vi "PowerGenerated.vi"() -> ()   [LabVIEW 2009]
uses:
  SubVis/Location.ctl
  <vilib>/Utility/file.llb/Read From Spreadsheet File (DBL).vi
  <vilib>/Analysis/NI_AALBase.lvlib
panel:
  out "Day of Max Power":i32 caption="Day:"
  out "Max Power":dbl caption="Max Power:" format="%#_3pW"
  in  "Location":T1
  out "Max Power (watts)":dbl(slide) caption="2.1MW" scale=0.0..40000000.0 scale format="%#_6pW"
  in  "Stop":bool
  in  "USA":bool
  in  "CostaRica":bool
  in  "Brazil":bool
  in  "India":bool
  in  "Australia":bool
  in  "Japan":bool
  in  "SouthAfrica":bool
  in  "Israel":bool
  in  "Germany":bool
  in  "Days of Month":u8(slide)=30 min=1 max=30 step=1 scale=1.0..30.0
  out "USA_Select":u16(ring)
  out "Germany_Select":u16(ring)
  out "Brazil_Select":u16(ring)
  out "Israel_Select":u16(ring)
  out "India_Select":u16(ring)
  out "Japan_Select":u16(ring)
  out "SouthAfrica_Select":u16(ring)
  out "Australia_Select":u16(ring)
  out "CostaRica_Select":u16(ring)
  out "Wind Speed of All Countries":waveform(dbl)[](graph)
  out "Power Per Country":dbl[](graph)
  # "The day of maximum power output for a given location is determined for all days starting from the first day of the month until the selected day. The power output and corresponding day are displayed numerically and the power output is also displayed on a meter."
  # "Choose the location and day of the month that you would like to be displayed on the Power Per Country graph. All data from the first day of the month up until the selected day will be displayed."
  # "All countries wind speed data over 30 days is displayed on this graph."
  # "TO DO:  \nWind plot gets thicker when country is selected.\nTips slide down from above in semitransparent window."
  # "40MW"
  # "MAX POWER:"
  # "Move the mouse over included countried to see a plot of their power generation capabilities.  The windspeed for the selected county is highlighted in the graph at the lower right.  \n\nThe  Max Power can be viewed in the top right indicator and graphically on the meter at the far right.  The peak Day appears as a dotted line.\n\nThe slide control above selects how many days in the month are viewed."
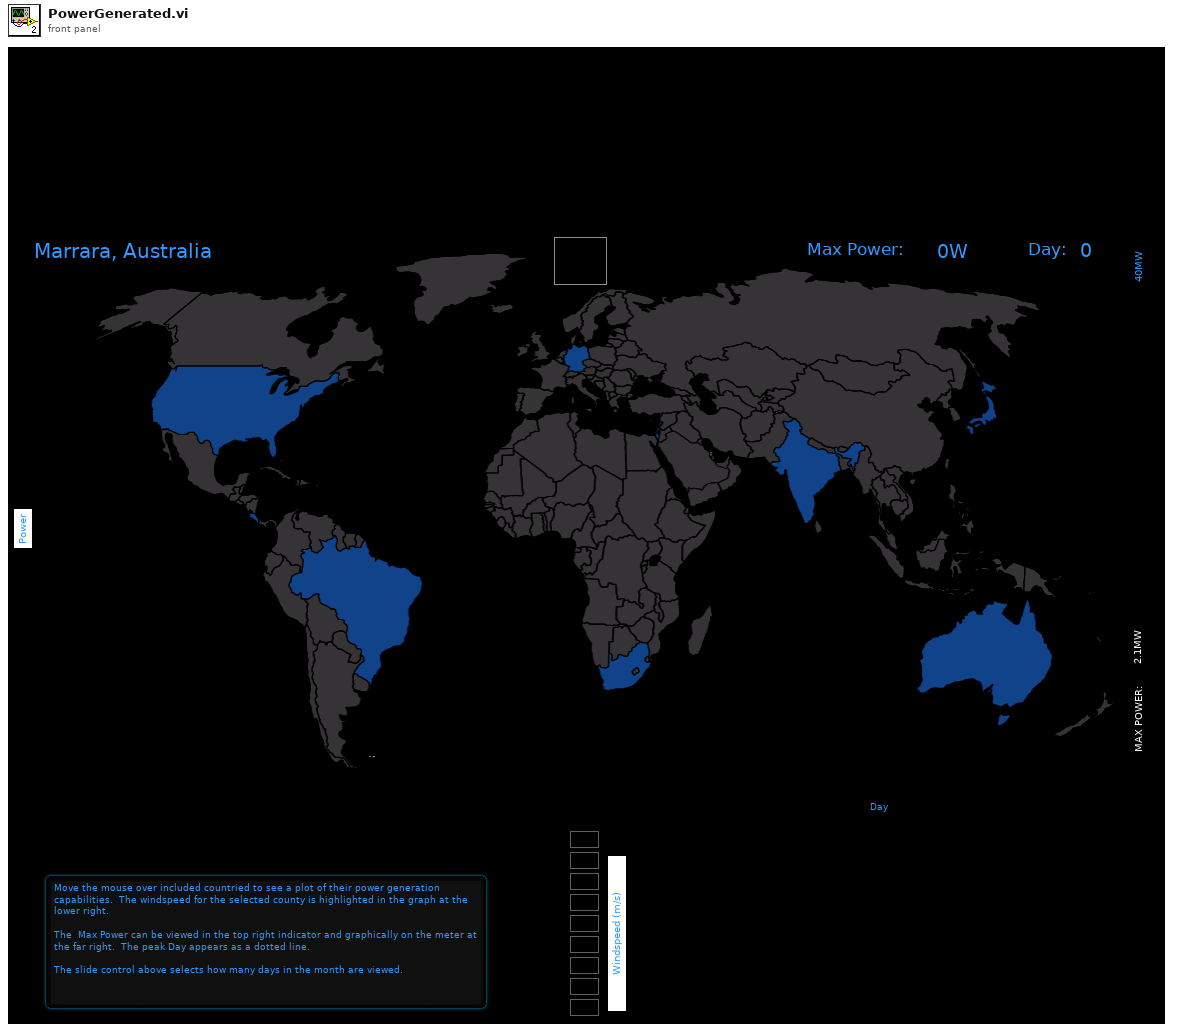
[diagram p1: front panel]
types:
  T1 = typedef "Location.ctl" = enum16{"Marrara, Australia", "Brasilia, Brazil", "Puerto Limon, Costa Rica", "Berlin, Germany", "Mumbai, India", "Sde-Dov, Israel", "Ise Bay, Japan", "Cape Good Hope, South Africa", "Texas, USA"}
  T2 = cluster{"Name":string, "Color":u32, "Style":u8, "Point Style":u8, "Name Visible":bool, "Allow Drag":bool, "Cursor Mode":u32, "Plot":i32, "Index":i32, "Position":cluster{"X":i32, "Y":i32}, "X Scale":u32, "Y Scale":u32, "Watch Plots":i32[], "Watch All Plots":bool, "Plot Area":i32, "Label Offset":cluster{"X":dbl, "Y":dbl}}
  T3 = cluster{"Name":string, "Color":u32, "Style":u8, "Point Style":u8, "Name Visible":bool, "Allow Drag":bool, "Annotation Mode":u32, "Plot":i32, "Index":i32, "Position":cluster{"X":dbl, "Y":dbl}, "X Scale":u32, "Y Scale":u32, "Show Arrow":bool, "Lock Name":bool, "Plot Area":i32, "Label Offset":cluster{"X":dbl, "Y":dbl}}
  T4 = cluster{"Location":T1, "Max Power":dbl, "Days of Month":u8, "Power Per Country":dbl[], "Day of Max Power":i32}
  T5 = cluster{"Name":string, "Color":u32, "Style":u8, "Point Style":u8, "Name Visible":bool, "Allow Drag":bool, "Annotation Mode":u32, "Plot":i32, "Index":i32, "Position":cluster{"X":dbl, "Y":dbl}, "X Scale":u32, "Y Scale":u32, "Show Arrow":bool, "Lock Name":bool, "Plot Area":i32, "Label Offset":cluster{"X":dbl, "Y":dbl}}[]
  T6 = cluster{"Name":string, "Color":u32, "Style":u8, "Point Style":u8, "Name Visible":bool, "Allow Drag":bool, "Cursor Mode":u32, "Plot":i32, "Index":i32, "Position":cluster{"X":i32, "Y":i32}, "X Scale":u32, "Y Scale":u32, "Watch Plots":i32[], "Watch All Plots":bool, "Plot Area":i32, "Label Offset":cluster{"X":dbl, "Y":dbl}}[]
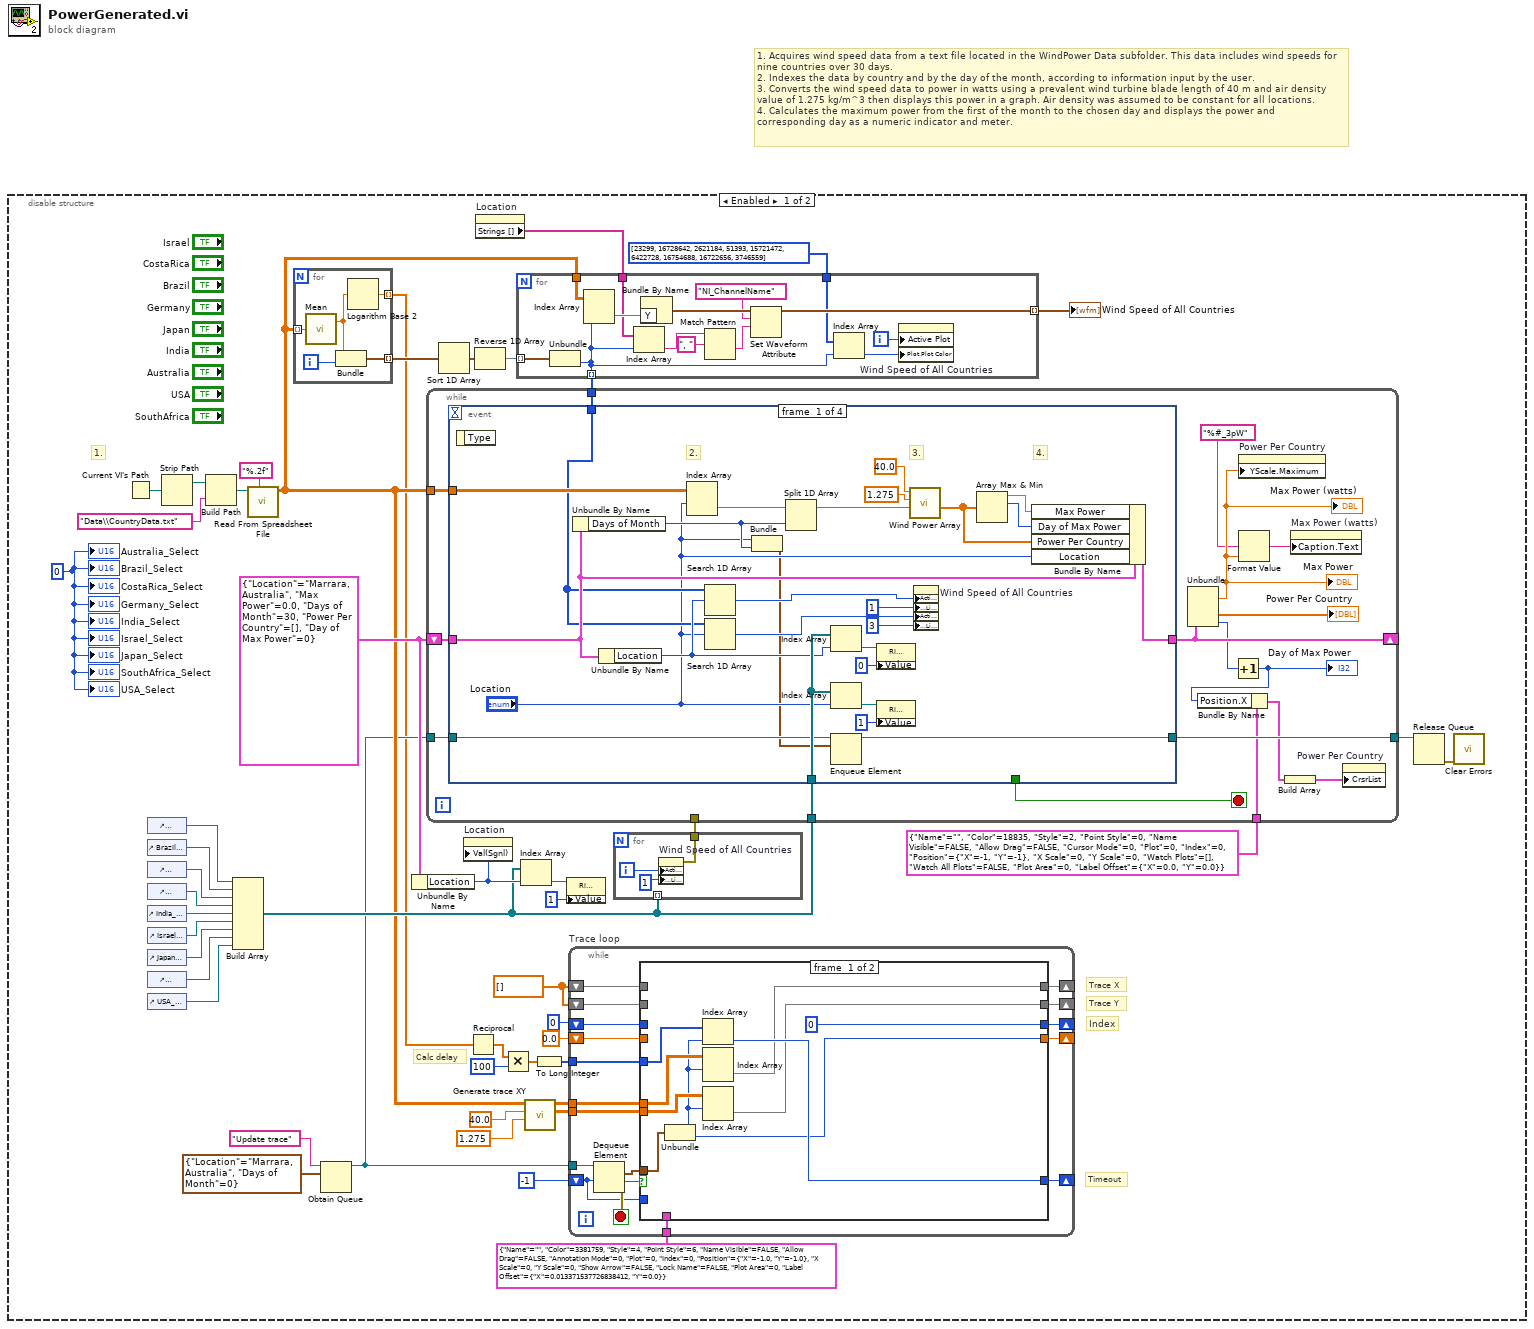
[diagram p0: block diagram]
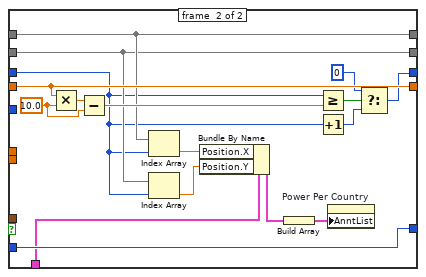
[diagram p2: hidden frame]
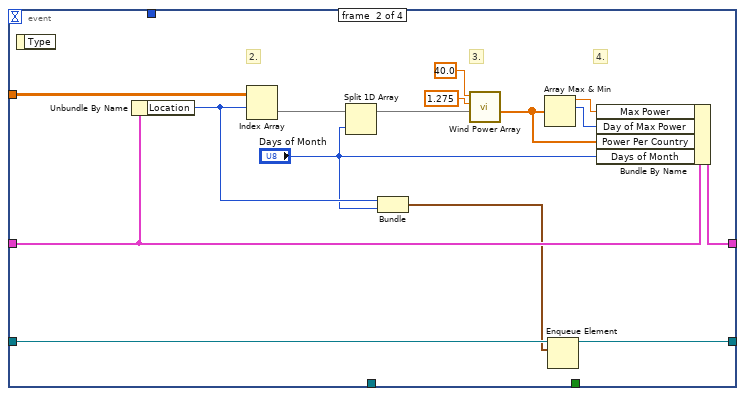
[diagram p3: hidden frame]
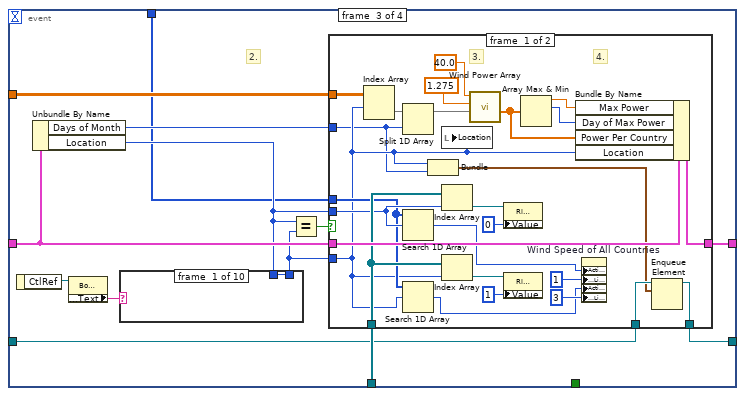
[diagram p4: hidden frame]
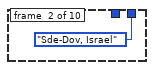
[diagram p6: hidden frame]
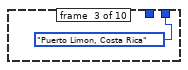
[diagram p7: hidden frame]
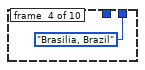
[diagram p8: hidden frame]
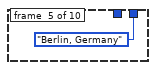
[diagram p9: hidden frame]
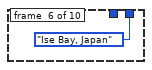
[diagram p10: hidden frame]
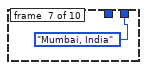
[diagram p11: hidden frame]
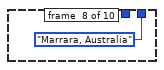
[diagram p12: hidden frame]
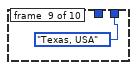
[diagram p13: hidden frame]
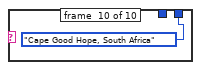
[diagram p14: hidden frame]
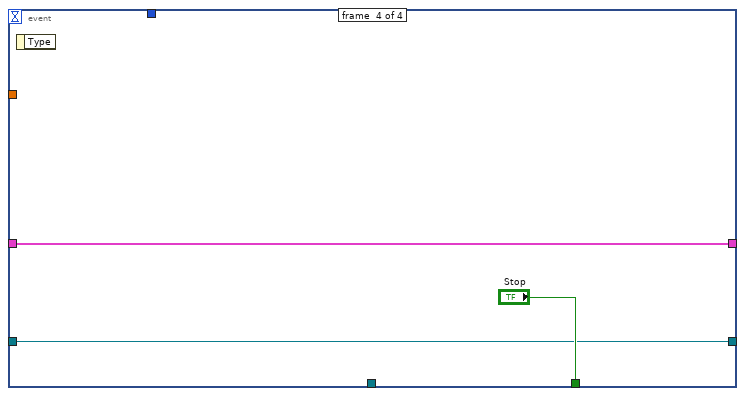
[diagram p15: hidden frame]
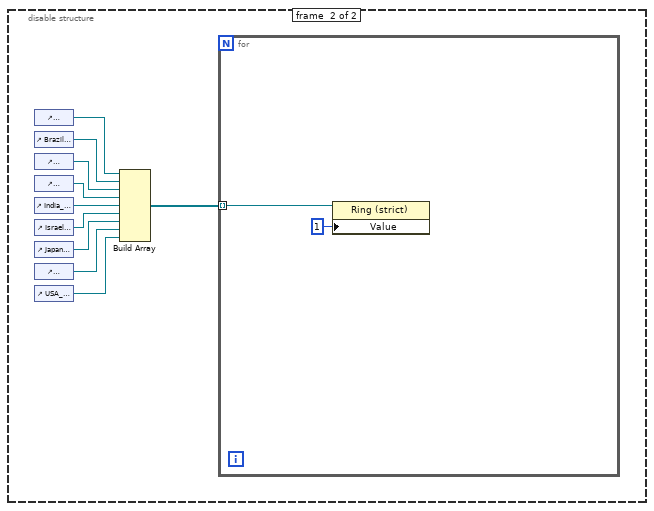
[diagram p16: hidden frame]
diagram:
  # "1. Acquires wind speed data from a text file located in the WindPower Data subfolder. This data includes wind speeds for nine countries over 30 days.\n2. Indexes the data by country and by the day of the month, according to information input by the user.\n3. Converts the wind speed data to power in watts using a prevalent wind turbine blade length of 40 m and air density value of 1.275 kg/m^3 then displays this power in a graph. Air density was assumed to be constant for all locations.\n4. Calculates the maximum power from the first of the month to the chosen day and displays the power and corresponding day as a numeric indicator and meter."
  n1 = disable-structure shown="Enabled" {
    frame #0 {
      w10 = dbl[] [] ("Trace X")
      w44 = u16 0 ("Japan_Select")
      w32 = T4 {"Location"=enum."Marrara, Australia", "Max Power"=0.0, "Days of Month"=30, "Power Per Country"=[], "Day of Max Power"=0}
      # "Index"
      # "Timeout"
      # "Trace Y"
      # "Trace X"
      # "Calc delay"
      # "1."
      n2 = Current VI's Path() -> (path=w48:path)
      n3 = control-ref of="Australia_Select"() -> (w43:refnum<vi>)
      n4 = control-ref of="Brazil_Select"() -> (w42:refnum<vi>)
      n5 = control-ref of="CostaRica_Select"() -> (w41:refnum<vi>)
      n6 = control-ref of="Germany_Select"() -> (w40:refnum<vi>)
      n7 = control-ref of="India_Select"() -> (w39:refnum<vi>)
      n8 = control-ref of="Israel_Select"() -> (w38:refnum<vi>)
      n9 = control-ref of="Japan_Select"() -> (w37:refnum<vi>)
      n10 = control-ref of="SouthAfrica_Select"() -> (w36:refnum<vi>)
      n11 = control-ref of="USA_Select"() -> (w35:refnum<vi>)
      n12 = Strip Path(path=w48) -> (stripped path=w47:path)  [unwired: 1 out]
      n13 = Build Path(base path=w47, name or relative path="Data\\CountryData.txt") -> (appended path=w46:path)
      n14 = Build Array(w43, w42, w41, w40, w39, w38, w37, w36, w35) -> (w23:refnum<vi>[])
      n15 = call-poly <vilib>:"Read From Spreadsheet File.vi"("format (%.3f)"="%.2f", "file path (dialog if empty)"=w46) -> ("all rows"=w21:dbl[][])  [unwired: 5 in, 4 out]
      n16 = for {
        tunnel: w21 -> [w113] mode=indexing
        tunnel: [w111] -> w30 mode=indexing
        tunnel: [w109] -> w2 mode=indexing
        i -> [w112]
        n17 = call <vilib>:"Mean.vi"("X"=w113) -> ("mean"=w110:dbl)  [unwired: 1 out]
        n18 = Bundle("mean"=w110, w112) -> (w111:cluster{"mean":dbl, i32})  [unwired: 1 in]
        n19 = Logarithm Base 2(1:w110) -> (0:w109:dbl)
      }
      n20 = Obtain Queue(name (unnamed)="Update trace", element data type=cluster{"Location":T1, "Days of Month":u8} {"Location"=enum."Marrara, Australia", "Days of Month"=0} ("cluster")) -> (queue out=w6:refnum<queue>)  [unwired: 3 in, 2 out]
      n21 = Unbundle By Name(w32) -> ("Location"=w31:T1)
      n22 = Sort 1D Array(array=w30) -> (sorted array=w27:cluster{"mean":dbl, i32}[])
      n23 = property on="Location" class="Enum (strict)"("Val(Sgnl)"=w31) -> ()  [unwired: 2 in, 2 out]
      n24 = Reciprocal(x=w2) -> (1/x=w3:dbl[])
      n25 = Reverse 1D Array(array=w27) -> (reversed array=w26:cluster{"mean":dbl, i32}[])
      n26 = property on="Location" class="Enum (strict)"() -> ("Strings []"=w28:string[])  [unwired: 2 in, 2 out]
      n27 = Multiply(x=w3, y=100 ("Numeric")) -> (x*y=w15:dbl[])
      n28 = for {
        tunnel: w26 -> [w108] mode=indexing
        tunnel: w21 -> [w107]
        tunnel: [w96] -> w25 mode=indexing
        tunnel: [w104] -> w29 mode=indexing
        tunnel: w28 -> [w102]
        tunnel: u32[] [23299, 16728642, 2621184, 51393, 15721472, 6422728, 16754688, 16722656, 3746559] ("Array") -> [w97]
        i -> [w98]
        n29 = Unbundle(w108) -> (w96:i32)  [unwired: 1 out]
        n30 = Index Array(array=w107, index (row)=w96) -> (element=w106:dbl[])  [unwired: 1 in]
        n31 = Index Array(array=w102, index=w96) -> (element=w100:string)
        n32 = Bundle By Name("Y"=w106) -> (w105:waveform(dbl))  [unwired: 1 in]
        n33 = Match Pattern(string=w100, regular expression=", ") -> (after substring=w99:string)  [unwired: 1 in, 3 out]
        n34 = Set Waveform Attribute(5:w99, 6:"NI_ChannelName" ("name"), 7:w105) -> (3:w104:waveform(dbl))  [unwired: 1 in, 2 out]
        n35 = Index Array(array=w97, index=w96) -> (element=w95:u32)
        n36 = property on="Wind Speed of All Countries" class="WFGraph (strict)"("Active Plot"=w98, "Plot.Plot Color"=w95) -> ()  [unwired: 2 in, 2 out]
      }
      "Wind Speed of All Countries" <- w29
      n37 = Index Array(array=w23, index=w31) -> (element=w33:refnum<vi>)
      n38 = call "Generate trace XY.vi"("Density"=1.275, "Blade Lenth"=40.0, "Windspeeds"=w21) -> ("Trace Y"=w12:dbl[][], "Trace X"=w13:dbl[][])  [unwired: 7 in]
      n39 = To Long Integer(number=w15) -> (32bit integer=w14:i32[])
      n40 = property class="Ring (strict)"(reference=w33, "Value"=u16 1) -> ()  [unwired: 1 in, 2 out]
      n41 = while "Trace loop" {
        tunnel: w6 -> [w67]
        tunnel: w14 -> [w61]
        tunnel: w13 -> [w63]
        tunnel: w12 -> [w62]
        shift-right: [w60] -> _
        shift-left: -1 ("timeout in ms (-1)") -> [w55]
        shift-right: [w59] -> _
        shift-left: w10 -> [w58]
        shift-right: [w56] -> _
        shift-left: w10 -> [w57]
        shift-right: [w54] -> _
        shift-left: 0 ("element") -> [w52]
        shift-right: [w53] -> _
        shift-left: 0.0 ("Days of Month") -> [w51]
        tunnel: T3 {"Name"="", "Color"=3381759, "Style"=4, "Point Style"=6, "Name Visible"=FALSE, "Allow Drag"=FALSE, "Annotation Mode"=0, "Plot"=0, "Index"=0, "Position"={"X"=-1.0, "Y"=-1.0}, "X Scale"=0, "Y Scale"=0, "Show Arrow"=FALSE, "Lock Name"=FALSE, "Plot Area"=0, "Label Offset"={"X"=0.013371537726838412, "Y"=0.0}} -> [w50]
        stop <- w66 stop-if-true
        n42 = Dequeue Element(queue=w67, timeout in ms (-1)=w55) -> (element=w64:cluster{"Location":T1, "Days of Month":u8}, timed out?=w65:bool, error out=w66:errorcluster)  [unwired: 1 in, 1 out]
        n43 = case shown="True" w65 {
          tunnel: w64 -> [w77 _]
          tunnel: w63 -> [w75 _]
          tunnel: w62 -> [w76 _]
          tunnel: w61 -> [w73 _]
          tunnel: [w72 w94] -> w60
          tunnel: w55 -> [_ w94]
          tunnel: [w71 w81] -> w59
          tunnel: w58 -> [_ w81]
          tunnel: w57 -> [_ w80]
          tunnel: [w70 w80] -> w56
          tunnel: [0 ("element") w86] -> w54
          tunnel: [w68 w93] -> w53
          tunnel: w52 -> [_ w78]
          tunnel: w51 -> [_ w93]
          tunnel: w50 -> [_ w83]
          frame #0 {
            n44 = Unbundle(w77) -> ("Location"=w74:T1, "Days of Month"=w68:u8)
            n45 = Index Array(array=w73, index=w74) -> (element=w72:i32)
            n46 = Index Array(array=w75, index (row)=w74) -> (element=w71:dbl[])  [unwired: 1 in]
            n47 = Index Array(array=w76, index (row)=w74) -> (element=w70:dbl[])  [unwired: 1 in]
          }
          frame #1 {
            w91 = 10.0 ("y")
            n48 = Multiply(x=w93, y=w91) -> (x*y=w92:dbl)
            n49 = Subtract(x=w92, y=w91) -> (x-y=w90:dbl)
            n50 = Index Array(array=w81, index=w78) -> (element=w82:dbl)
            n51 = Index Array(array=w80, index=w78) -> (element=w79:dbl)
            n52 = Bundle By Name(cluster=w83, "Position.X"=w82, "Position.Y"=w79) -> (w84:T3)
            n53 = Build Array(w84) -> (w85:T5)
            n54 = Greater Or Equal?(x=w78, y=w90) -> (x >= y?=w89:bool)
            n55 = Increment(x=w78) -> (x+1=w88:i32)
            n56 = property on="Power Per Country" class="WFGraph (strict)"("AnntList"=w85) -> ()  [unwired: 2 in, 2 out]
            n57 = Select(t=0, s=w89, f=w88) -> (s? t:f=w86:i32)
          }
        }
      }
      n58 = for {
        tunnel: w23 -> [_] mode=indexing
        tunnel: [w114] -> w22
        i -> [w116]
        n59 = property on="Wind Speed of All Countries" class="WFGraph (strict)"("Active Plot"=w116, "Plot.Line Width"=u8 1 ("f")) -> (error out=w114:errorcluster)  [unwired: 2 in, 1 out]
      }
      n60 = while {
        tunnel: w21 -> [w133]
        shift-right: [w130] -> _
        shift-left: w32 -> [w131]
        tunnel: w23 -> [w127]
        tunnel: w25 -> [w126]
        tunnel: w22 -> [_]
        tunnel: w6 -> [w122]
        tunnel: [w121] -> w5
        tunnel: T2 {"Name"="", "Color"=18835, "Style"=2, "Point Style"=0, "Name Visible"=FALSE, "Allow Drag"=FALSE, "Cursor Mode"=0, "Plot"=0, "Index"=0, "Position"={"X"=-1, "Y"=-1}, "X Scale"=0, "Y Scale"=0, "Watch Plots"=[], "Watch All Plots"=FALSE, "Plot Area"=0, "Label Offset"={"X"=0.0, "Y"=0.0}} ("element") -> [w119]
        stop <- w132 stop-if-true
        n61 = event shown="[1] \"Days of Month\": Value Change" {
          selector: _ -> [_ _ _ _]
          dyn-events: _ -> [_ _ _ _]
          timeout: _ -> [_ _ _ _]
          tunnel: w133 -> [w159 w170 w185 _]
          tunnel: [_ _ _ "Stop"] -> w132
          tunnel: w131 -> [w145 w168 w183 w227]
          tunnel: [w151 w169 w182 w227] -> w130
          tunnel: w127 -> [w146 _ w181 _]
          tunnel: w126 -> [w140 _ w177 _]
          tunnel: w122 -> [w136 w164 w176 w226]
          tunnel: [w134 w163 w175 w226] -> w121
          event #0 {
            # "4."
            # "3."
            # "2."
            n62 = event-data() -> ()  [unwired: 1 in, 1 out]
            n63 = Unbundle By Name(w145) -> ("Days of Month"=w138:u8)
            n64 = Unbundle By Name(w145) -> ("Location"=w142:T1)
            n65 = Index Array "Index Array"(array=w159, index (row)="Location") -> (element=w156:dbl[])  [unwired: 1 in]
            n66 = Search 1D Array(1D array=w140, element=w142) -> (index of element=w141:i32)  [unwired: 1 in]
            n67 = Search 1D Array(1D array=w140, element="Location") -> (index of element=w139:i32)  [unwired: 1 in]
            n68 = Bundle("Location"="Location", "Days of Month"=w138) -> (w135:cluster{"Location":T1, "Days of Month":u8})  [unwired: 1 in]
            n69 = Split 1D Array(array=w156, index=w138) -> (first subarray=w155:dbl[])  [unwired: 1 out]
            n70 = Index Array(array=w146, index=w142) -> (element=w150:refnum<vi>)
            n71 = Index Array(array=w146, index="Location") -> (element=w148:refnum<vi>)
            n72 = Enqueue Element(queue=w136, element=w135) -> (queue out=w134:refnum<queue>)  [unwired: 2 in, 2 out]
            n73 = property class="Ring (strict)"(reference=w150, "Value"=u16 0) -> ()  [unwired: 1 in, 2 out]
            n74 = property class="Ring (strict)"(reference=w148, "Value"=u16 1) -> ()  [unwired: 1 in, 2 out]
            n75 = call "Wind Power Array.vi"("Wind Speed (m/s)"=w155, "Density (kg/m^3)"=1.275 ("Density"), "Blade Length (m)"=40.0 ("Blade Lenth")) -> ("Power (watts)"=w154:dbl[])  [unwired: 8 in]
            n76 = property on="Wind Speed of All Countries" class="WFGraph (strict)"("Active Plot"=w141, "Plot.Line Width"=u8 1, "Active Plot"=w139, "Plot.Line Width"=u8 3) -> ()  [unwired: 2 in, 2 out]
            n77 = Array Max & Min(array=w154) -> (max value=w153:dbl, max index (indices)=w152:i32)  [unwired: 2 out]
            n78 = Bundle By Name(cluster=w145, "Max Power"=w153, "Day of Max Power"=w152, "Power Per Country"=w154, "Location"="Location") -> (w151:T4)
          }
          event #1 {
            # "4."
            # "3."
            # "2."
            n79 = event-data() -> ()  [unwired: 1 in, 1 out]
            n80 = Unbundle By Name(w168) -> ("Location"=w162:T1)
            n81 = Index Array "Index Array"(array=w170, index (row)=w162) -> (element=w172:dbl[])  [unwired: 1 in]
            n82 = Split 1D Array(array=w172, index="Days of Month") -> (first subarray=w171:dbl[])  [unwired: 1 out]
            n83 = Bundle("Location"=w162, "Days of Month"="Days of Month") -> (w160:cluster{"Location":T1, "Days of Month":u8})  [unwired: 1 in]
            n84 = call "Wind Power Array.vi"("Wind Speed (m/s)"=w171, "Density (kg/m^3)"=1.275 ("Density"), "Blade Length (m)"=40.0 ("Blade Lenth")) -> ("Power (watts)"=w167:dbl[])  [unwired: 8 in]
            n85 = Array Max & Min(array=w167) -> (max value=w166:dbl, max index (indices)=w165:i32)  [unwired: 2 out]
            n86 = Enqueue Element(queue=w164, element=w160) -> (queue out=w163:refnum<queue>)  [unwired: 2 in, 2 out]
            n87 = Bundle By Name(cluster=w168, "Max Power"=w166, "Day of Max Power"=w165, "Power Per Country"=w167, "Days of Month"="Days of Month") -> (w169:T4)
          }
          event #2 {
            # "2."
            n88 = event-data() -> ("CtlRef"=w187:refnum<vi>)  [unwired: 1 in]
            n89 = Unbundle By Name(w183) -> ("Days of Month"=w184:u8, "Location"=w180:T1)
            n90 = property class="Bool (strict)"(reference=w187) -> ("Label.Text"=w186:string)  [unwired: 1 in, 2 out]
            n91 = case shown="\"Germany\"" w186 {
              tunnel: [w216 Location."Sde-Dov, Israel" ("Location") Location."Puerto Limon, Costa Rica" ("Location") Location."Brasilia, Brazil" ("Location") Location."Berlin, Germany" ("Location") Location."Ise Bay, Japan" ("Location") Location."Mumbai, India" ("Location") Location."Marrara, Australia" ("Location") Location."Texas, USA" ("Location") Location."Cape Good Hope, South Africa" ("Location")] -> w179
              tunnel: w180 -> [w216 _ _ _ _ _ _ _ _ _]
              frame #0 {
              }
              frame #1 {
              }
              frame #2 {
              }
              frame #3 {
              }
              frame #4 {
              }
              frame #5 {
              }
              frame #6 {
              }
              frame #7 {
              }
              frame #8 {
              }
              frame #9 {
              }
            }
            n92 = Equal?(x=w180, y=w179) -> (x = y?=w178:bool)
            n93 = case shown="True" w178 {
              tunnel: w185 -> [w209 _]
              tunnel: w184 -> [w189 _]
              tunnel: w183 -> [w205 w215]
              tunnel: [w204 w215] -> w182
              tunnel: w181 -> [w203 _]
              tunnel: w180 -> [w194 _]
              tunnel: w179 -> [w190 _]
              tunnel: w177 -> [w193 _]
              tunnel: w176 -> [w192 w214]
              tunnel: [w191 w214] -> w175
              frame #0 {
                # "4."
                # "3."
                n94 = Index Array(array=w209, index (row)=w190) -> (element=w211:dbl[])  [unwired: 1 in]
                n95 = Split 1D Array(array=w211, index=w189) -> (first subarray=w210:dbl[])  [unwired: 1 out]
                n96 = Search 1D Array(1D array=w193, element=w194) -> (index of element=w196:i32)  [unwired: 1 in]
                n97 = Search 1D Array(1D array=w193, element=w190) -> (index of element=w195:i32)  [unwired: 1 in]
                n98 = Bundle("Location"=w190, "Days of Month"=w189) -> (w188:cluster{"Location":T1, "Days of Month":u8})  [unwired: 1 in]
                n99 = local write "Location"(w190) -> ()
                n100 = Index Array(array=w203, index=w194) -> (element=w202:refnum<vi>)
                n101 = Index Array(array=w203, index=w190) -> (element=w200:refnum<vi>)
                n102 = call "Wind Power Array.vi"("Wind Speed (m/s)"=w210, "Density (kg/m^3)"=1.275 ("Density"), "Blade Length (m)"=40.0 ("Blade Lenth")) -> ("Power (watts)"=w206:dbl[])  [unwired: 8 in]
                n103 = property class="Ring (strict)"(reference=w202, "Value"=u16 0) -> ()  [unwired: 1 in, 2 out]
                n104 = property class="Ring (strict)"(reference=w200, "Value"=u16 1) -> ()  [unwired: 1 in, 2 out]
                n105 = Array Max & Min(array=w206) -> (max value=w207:dbl, max index (indices)=w208:i32)  [unwired: 2 out]
                n106 = Bundle By Name(cluster=w205, "Max Power"=w207, "Day of Max Power"=w208, "Power Per Country"=w206, "Location"=w190) -> (w204:T4)
                n107 = property on="Wind Speed of All Countries" class="WFGraph (strict)"("Active Plot"=w196, "Plot.Line Width"=u8 1, "Active Plot"=w195, "Plot.Line Width"=u8 3) -> ()  [unwired: 2 in, 2 out]
                n108 = Enqueue Element(queue=w192, element=w188) -> (queue out=w191:refnum<queue>)  [unwired: 2 in, 2 out]
              }
              frame #1 {
              }
            }
          }
          event #3 {
            n109 = event-data() -> ()  [unwired: 1 in, 1 out]
          }
        }
        n110 = Unbundle(w130) -> ("Max Power"=w125:dbl, "Power Per Country"=→"Power Per Country":dbl[], "Day of Max Power"=w128:i32)  [unwired: 2 out]
        "Max Power" <- w125
        "Max Power (watts)" <- w125
        n111 = Increment(x=w128) -> (x+1=w118:i32)
        "Day of Max Power" <- w118
        n112 = Bundle By Name(cluster=w119, "Position.X"=w118) -> (w117:T2)
        n113 = property on="Power Per Country" class="WFGraph (strict)"("YScale.Maximum"=w125) -> ()  [unwired: 2 in, 2 out]
        n114 = Format Value(format string="%#_3pW", value (0)=w125) -> (output string=w123:string)  [unwired: 1 in]
        n115 = Build Array(w117) -> (w120:T6)
        n116 = property on="Max Power (watts)" class="Slide (strict)"("Caption.Text"=w123) -> ()  [unwired: 2 in, 2 out]
        n117 = property on="Power Per Country" class="WFGraph (strict)"("CrsrList"=w120) -> ()  [unwired: 2 in, 2 out]
      }
      n118 = Release Queue(queue=w5) -> (error out=w4:errorcluster)  [unwired: 2 in, 2 out]
      n119 = call <vilib>:"Clear Errors.vi"("error in (no error)"=w4) -> ()  [unwired: 6 in, 1 out]
      "USA_Select" <- w44
      "CostaRica_Select" <- w44
      "Israel_Select" <- w44
      "Germany_Select" <- w44
      "India_Select" <- w44
      "Australia_Select" <- w44
      "Brazil_Select" <- w44
      "Japan_Select" <- w44
      "SouthAfrica_Select" <- w44
    }
    frame #1 {
      n120 = control-ref of="Australia_Select"() -> (w238:refnum<vi>)
      n121 = control-ref of="Brazil_Select"() -> (w237:refnum<vi>)
      n122 = control-ref of="CostaRica_Select"() -> (w236:refnum<vi>)
      n123 = control-ref of="Germany_Select"() -> (w235:refnum<vi>)
      n124 = control-ref of="India_Select"() -> (w234:refnum<vi>)
      n125 = control-ref of="Israel_Select"() -> (w233:refnum<vi>)
      n126 = control-ref of="Japan_Select"() -> (w232:refnum<vi>)
      n127 = control-ref of="SouthAfrica_Select"() -> (w231:refnum<vi>)
      n128 = control-ref of="USA_Select"() -> (w230:refnum<vi>)
      n129 = Build Array(w238, w237, w236, w235, w234, w233, w232, w231, w230) -> (w229:refnum<vi>[])
      n130 = for {
        tunnel: w229 -> [w240] mode=indexing
        n131 = property class="Ring (strict)"(reference=w240, "Value"=u16 1) -> ()  [unwired: 1 in, 2 out]
      }
    }
  }
